vi "Process.vi"(8 "error in (no error)":errorcluster, 10 "Pound in":refnum<class "Pound.lvclass">, 11 "Qbus in":refnum<class "Qbus.lvclass">) -> (0 "error out":errorcluster)   [LabVIEW 2017, in "McsaModbusMaster.lvlib"]
uses:
  <vilib>/addons/InsightCM/Devices/Shared/Mcsa/McsaModbusMaster/McsaModbusMaster.lvlib
  <vilib>/addons/Qbus/Qbus.lvclass
  <vilib>/NI/Software Watchdog/Pound/Pound.lvclass
  <vilib>/addons/InsightCM/Devices/Shared/Common/ModbusMaster/controls/config.ctl
  <vilib>/addons/InsightCM/Devices/Shared/Common/ModbusMaster/controls/ModbusDevice.ctl
  <vilib>/Modbus/master/Modbus Master.lvclass
  <vilib>/addons/InsightCM/Devices/Shared/Common/ModbusMaster/controls/ModbusChannel.ctl
  <vilib>/addons/InsightCM/Devices/Shared/Common/ModbusMaster/controls/RegisterType.ctl
  <vilib>/addons/InsightCM/MessageBus/Base/controls/DataSource.ctl
  <vilib>/addons/InsightCM/MessageBus/Base/controls/KeyValuePair.ctl
  <vilib>/addons/TraceLogger/TraceLogger.lvlib
  <vilib>/addons/InsightCM/Devices/Shared/Common/ModbusMaster/ModbusMaster.lvlib
  <vilib>/addons/InsightCM/Devices/Shared/Common/ServerComm/ServerComm.lvlib
  <vilib>/NI/Software Watchdog/Watchdog/Watchdog.lvclass
  <vilib>/addons/InsightCM/Utilities/GlobalConfiguration/GlobalConfiguration.lvlib
  <vilib>/addons/InsightCM/Utilities/PropertyHelpers/PropertyHelpers.lvlib
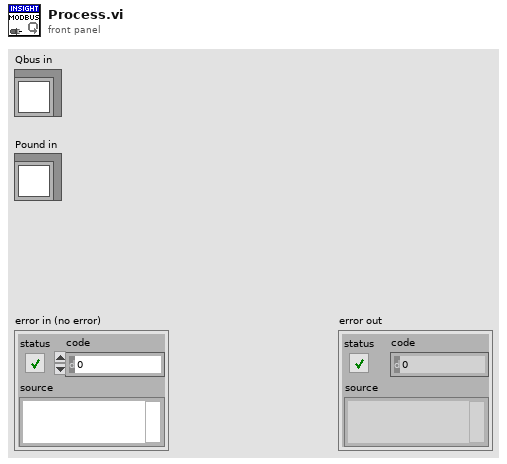
[diagram p1: front panel]
types:
  T1 = typedef "ModbusMaster.lvlib/config.ctl" = cluster{"Devices":T2[], "ReadTimeout":i32}
  T2 = typedef "ModbusMaster.lvlib/ModbusDevice.ctl" = cluster{"reference":refnum<class "Modbus Master.lvclass">, "Serial":bool, "ReadInterval (sec)":dbl, "ReadTimeout (ms)":i32, "LastRead":dbl, "channels":T3[], "connected":bool, "DataSource":T5}
  T3 = typedef "ModbusMaster.lvlib/ModbusChannel.ctl" = cluster{"RegisterType":T4, "Address":i32, "32bitRegister":bool, "FirstWordLow":bool, "Slope":dbl, "Offset":dbl, "ValueTag":string, "Name":string, "Range Check":bool, "MinimumEU":dbl, "MaximumEU":dbl, "Groups":string[]}
  T4 = typedef "ModbusMaster.lvlib/RegisterType.ctl" = enum16{"Unknown", "Coil", "Discrete Input", "Holding Register", "Input Register"}
  T5 = typedef "DataSource.ctl" = cluster{"Id":string, "Type":string, "Name":string, "MeasType":string, "Properties":T6[]}
  T6 = typedef "KeyValuePair.ctl" = cluster{"Key":string, "Value":string}
  T7 = typedef "SectionKeyValues.ctl" = cluster{"Section":string, "KeyValues":T6[]}
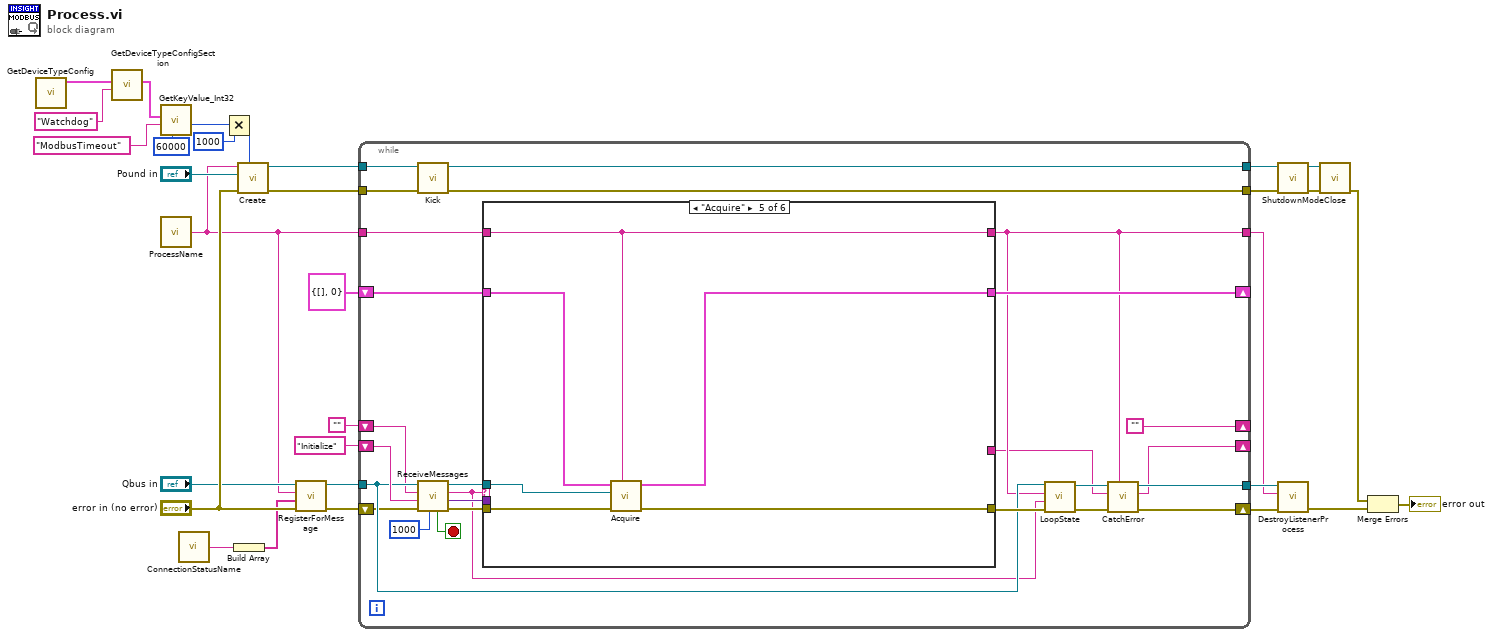
[diagram p0: block diagram]
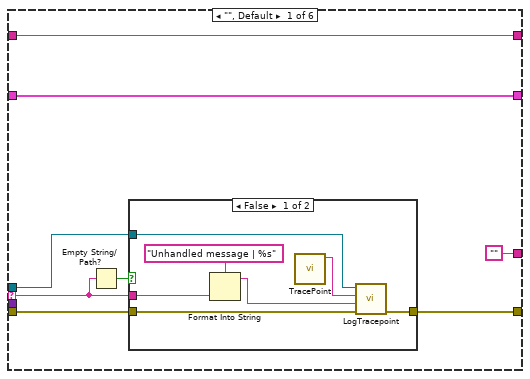
[diagram p2: hidden frame]
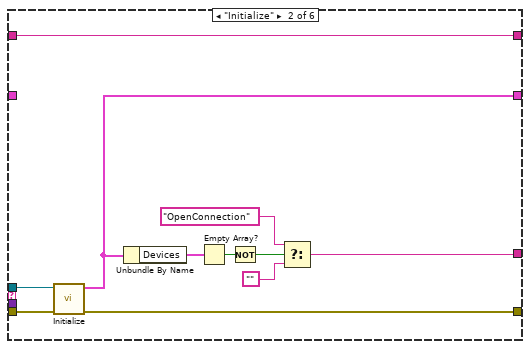
[diagram p4: hidden frame]
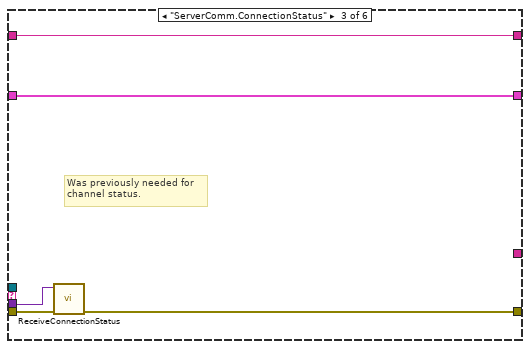
[diagram p5: hidden frame]
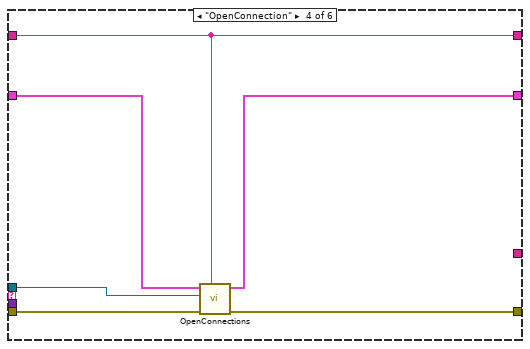
[diagram p6: hidden frame]
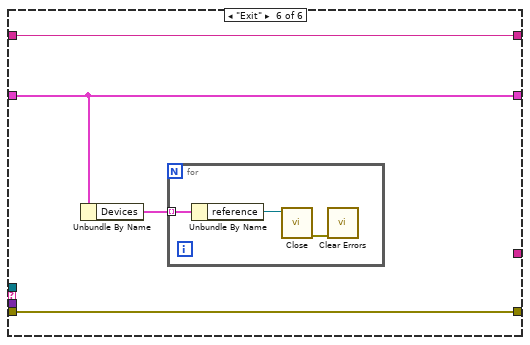
[diagram p7: hidden frame]
diagram:
  n1 = call <vilib>:"GetDeviceTypeConfig.vi"() -> ("key values"=w15:T7[])  [unwired: 9 in, 2 out]
  n2 = call <vilib>:"GetDeviceTypeConfigSection.vi"("key"="Watchdog", "key values"=w15) -> ("key value pairs out"=w12:T6[])  [unwired: 8 in, 1 out]
  n3 = call <vilib>:"GetKeyValue_Int32.vi"("default"=60000, "key"="ModbusTimeout" ("Tag"), "key value pairs"=w12) -> ("value"=w9:i32)  [unwired: 6 in, 2 out]
  n4 = call <vilib>:"ProcessName.vi"() -> ("process name"=w3:string)  [unwired: 5 in]
  n5 = call <vilib>:"ConnectionStatusName.vi"() -> ("message name"=w2:string)  [unwired: 5 in]
  n6 = Multiply(x=w9, y=1000) -> (x*y=w8:i32)
  n7 = Build Array(w2) -> (w1:string[])
  n8 = call <vilib>:"Create.vi"("Execution Timeout (ms)"=w8, "error in (no error)"="error in (no error)", "Pound"="Pound in", "Name"=w3) -> ("error out"=w20:errorcluster, "Watchdog"=w25:refnum<data-value>)  [unwired: 6 in]
  n9 = call <vilib>:"RegisterForMessage.vi"("error in (no error)"="error in (no error)", "message names"=w1, "process name"=w3, "Qbus in"="Qbus in") -> ("error in (no error)"=w6:errorcluster, "Qbus out"=w4:refnum<class "Qbus.lvclass">)  [unwired: 6 in]
  n10 = while {
    shift-right: [""] -> _
    shift-left: "" -> [w33]
    tunnel: w4 -> [w46]
    tunnel: w3 -> [w36]
    tunnel: [w49] -> w29
    tunnel: [w35] -> w28
    shift-right: [w48] -> _
    shift-left: "Initialize" -> [w53]
    shift-right: [w51] -> _
    shift-left: T1 {"Devices"=[], "ReadTimeout"=0} ("config") -> [w52]
    tunnel: w25 -> [w45]
    tunnel: [w44] -> w22
    tunnel: w20 -> [w43]
    tunnel: [w41] -> w19
    shift-right: [w50] -> w30
    shift-left: w6 -> [w42]
    stop <- w57 stop-if-true
    n11 = call <vilib>:"Kick.vi"("error in (no error)"=w43, "Watchdog"=w45) -> ("error out"=w41:errorcluster, "Watchdog"=w44:refnum<data-value>)  [unwired: 8 in]
    n12 = call <vilib>:"ReceiveMessages.vi"("Timeout(1000)"=1000 ("milliseconds to wait"), "error in (no error)"=w42, "priority action"=w53, "default action"=w33, "Qbus in"=w46) -> ("error out"=w56:errorcluster, "message value"=w54:variant, "action"=w40:string, "Qbus out"=w55:refnum<class "Qbus.lvclass">, "exit"=w57:bool)  [unwired: 2 in]
    n13 = case shown="\"Acquire\"" w40 {
      selector: w40 -> [w61 _ _ _ _ _]
      tunnel: w56 -> [w63 w82 w88 w95 w101 w105]
      tunnel: w55 -> [w59 w83 _ w92 w96 _]
      tunnel: [w62 w81 w87 w91 w98 w105] -> w47
      tunnel: w54 -> [_ _ w86 _ _ _]
      tunnel: w52 -> [w65 _ w85 w94 w100 w103]
      tunnel: [w65 w77 w85 w93 w99 w103] -> w51
      tunnel: [w64 w84 w89 w90 w97 w104] -> w35
      tunnel: w36 -> [w64 w84 w89 w90 w97 w104]
      tunnel: ["" w78 _ _ _ _] -> w34
      frame "", Default {
        n14 = Empty String/Path?(string/path=w61) -> (empty?=w60:bool)
        n15 = case shown="False" w60 {
          tunnel: [w69 w73] -> w62
          tunnel: w63 -> [w70 w73]
          tunnel: w61 -> [w72 _]
          tunnel: w59 -> [w68 _]
          frame False {
            n16 = Format Into String(format string="Unhandled message | %s", w72) -> (resulting string=w67:string)  [unwired: 2 in, 1 out]
            n17 = call <vilib>:"TracePoint.vi"() -> ("template trace point"=w66:string)  [unwired: 11 in]
            n18 = call <vilib>:"LogTracepoint.vi"("error in (no error)"=w70, "log string"=w67, "tracepoint"=w66, "qbus in"=w68) -> ("error out"=w69:errorcluster)  [unwired: 6 in, 1 out]
          }
          frame True {
          }
        }
      }
      frame "Initialize" {
        n19 = call <vilib>:"Initialize.vi"("error in (no error)"=w82, "Qbus"=w83) -> ("error out"=w81:errorcluster, "config"=w77:T1)  [unwired: 8 in]
        n20 = Unbundle By Name(w77) -> ("Devices"=w76:T2[])
        n21 = Empty Array?(array=w76) -> (empty?=w75:bool)
        n22 = Not(x=w75) -> (.not. x?=w74:bool)
        n23 = Select(t="OpenConnection", s=w74, f="") -> (s? t:f=w78:string)
      }
      frame "ServerComm.ConnectionStatus" {
        # "Was previously needed for\nchannel status."
        n24 = call <vilib>:"ReceiveConnectionStatus.vi"("error in (no error)"=w88, "body"=w86) -> ("error out"=w87:errorcluster)  [unwired: 6 in, 3 out]
      }
      frame "OpenConnection" {
        n25 = call <vilib>:"OpenConnections.vi"("process name"=w90, "error in (no error)"=w95, "Qbus"=w92, "config in"=w94) -> ("error out"=w91:errorcluster, "config out"=w93:T1)  [unwired: 6 in]
      }
      frame "Acquire" {
        n26 = call <vilib>:"Acquire.vi"("process name"=w97, "error in (no error)"=w101, "Qbus in"=w96, "config in"=w100) -> ("error out"=w98:errorcluster, "config out"=w99:T1)  [unwired: 6 in]
      }
      frame "Exit" {
        n27 = Unbundle By Name(w103) -> ("Devices"=w102:T2[])
        n28 = for {
          tunnel: w102 -> [w108] mode=indexing
          n29 = Unbundle By Name(w108) -> ("reference"=w107:refnum<class "Modbus Master.lvclass">)
          n30 = call-dynamic <vilib>:"Close.vi"("Modbus master in"=w107) -> ("error out"=w106:errorcluster)  [unwired: 10 in]
          n31 = call <vilib>:"Clear Errors.vi"("error in (no error)"=w106) -> ()  [unwired: 5 in, 2 out]
        }
      }
    }
    n32 = call <vilib>:"LoopState.vi"("error in (no error)"=w47, "loop action"=w40, "process name"=w35, "Qbus in"=w46) -> ("error out"=w38:errorcluster, "Qbus out"=w37:refnum<class "Qbus.lvclass">)  [unwired: 6 in]
    n33 = call <vilib>:"CatchError.vi"("source"=w35, "error in (no error)"=w38, "next action in"=w34, "Qbus in"=w37) -> ("error out"=w50:errorcluster, "next action out"=w48:string, "Qbus out"=w49:refnum<class "Qbus.lvclass">)  [unwired: 5 in]
  }
  n34 = call <vilib>:"ShutdownMode.vi"("error in (no error)"=w19, "Watchdog"=w22) -> ("error out"=w21:errorcluster, "Watchdog"=w23:refnum<data-value>)  [unwired: 8 in]
  n35 = call <vilib>:"DestroyListenerProcess.vi"("error in (no error)"=w30, "process name"=w28, "Qbus in"=w29) -> ("error in (no error)"=w18:errorcluster)  [unwired: 7 in, 1 out]
  n36 = call <vilib>:"Close.vi"("error in (no error)"=w21, "Watchdog"=w23) -> ("error out"=w17:errorcluster)  [unwired: 9 in]
  n37 = Merge Errors(w17, w18) -> (→"error out":errorcluster)
